vi "UI Limit Sensor.vi"(8 "error in":errorcluster) -> (0 "error out":errorcluster)   [LabVIEW 2019, in "Test.lvlib"]
uses:
  Test.lvlib
  Queues/Message Cluster.ctl
  Fluidic Process/SubVI/Fluidic Para.ctl
  <vilib>/Utility/file.llb/Write Delimited Spreadsheet (string).vi
  <vilib>/Utility/file.llb/Read Delimited Spreadsheet (string).vi
  Controller/Controller.lvlib
  Queues/Queues.lvlib
  Fluidic Process/Fluidic Process.lvlib
  Syringe Pump/NE-500/NE-500.lvlib
  Initialize/Initialize.lvlib
panel:
  out "Limit Sensor":bool
  in  "Stop Process":bool
  out "Remaining Time(s)":dbl
  out "Total Process":string
  out "Current Process":string
  out "Gauge":dbl(knob)=1.2869315802184793e-48 scale=0.0..100.0
  in  "Limit Sensor":bool
  in  "Back":bool
  # "/"
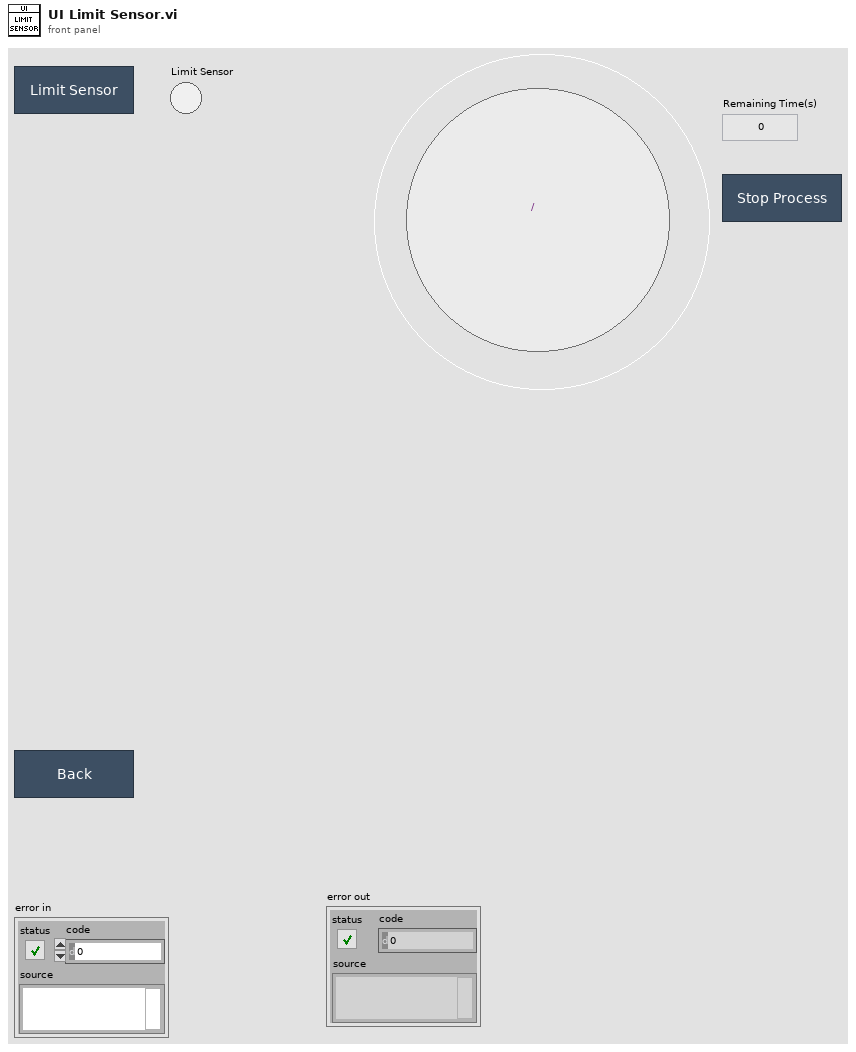
[diagram p1: front panel]
types:
  T1 = cluster{"Limit Sensor":refnum<queue>, "Limit Sensor Data":refnum<queue>}
  T2 = enum8{"Enabled", "Disabled", "Disabled and Grayed Out"}
  T3 = typedef "Fluidic Process.lvlib/Fluidic Para.ctl" = cluster{"Read Force Sensor":i32, "Read Regulator":i32, "Read Force Sensor?":bool, "Read Regulator?":bool, "Read Syringe Pump":i32, "Read Syringe Pump?":bool}
  T4 = typedef "Fluidic Process.lvlib/SEQ Data.ctl" = cluster{"Fluidic Process Done?":bool, "Current Process":i32, "Remaining Time":dbl, "Total Process":i32, "Air Sealing":bool, "Force Condition":bool}
  T5 = typedef "Initialize.lvlib/SEQ Data.ctl" = cluster{"Folder Path":path}
  T6 = typedef "NE-500.lvlib/SEQ Data.ctl" = cluster{"Status":string, "Initialize Done?":bool, "VI Refnum":refnum<vi>}
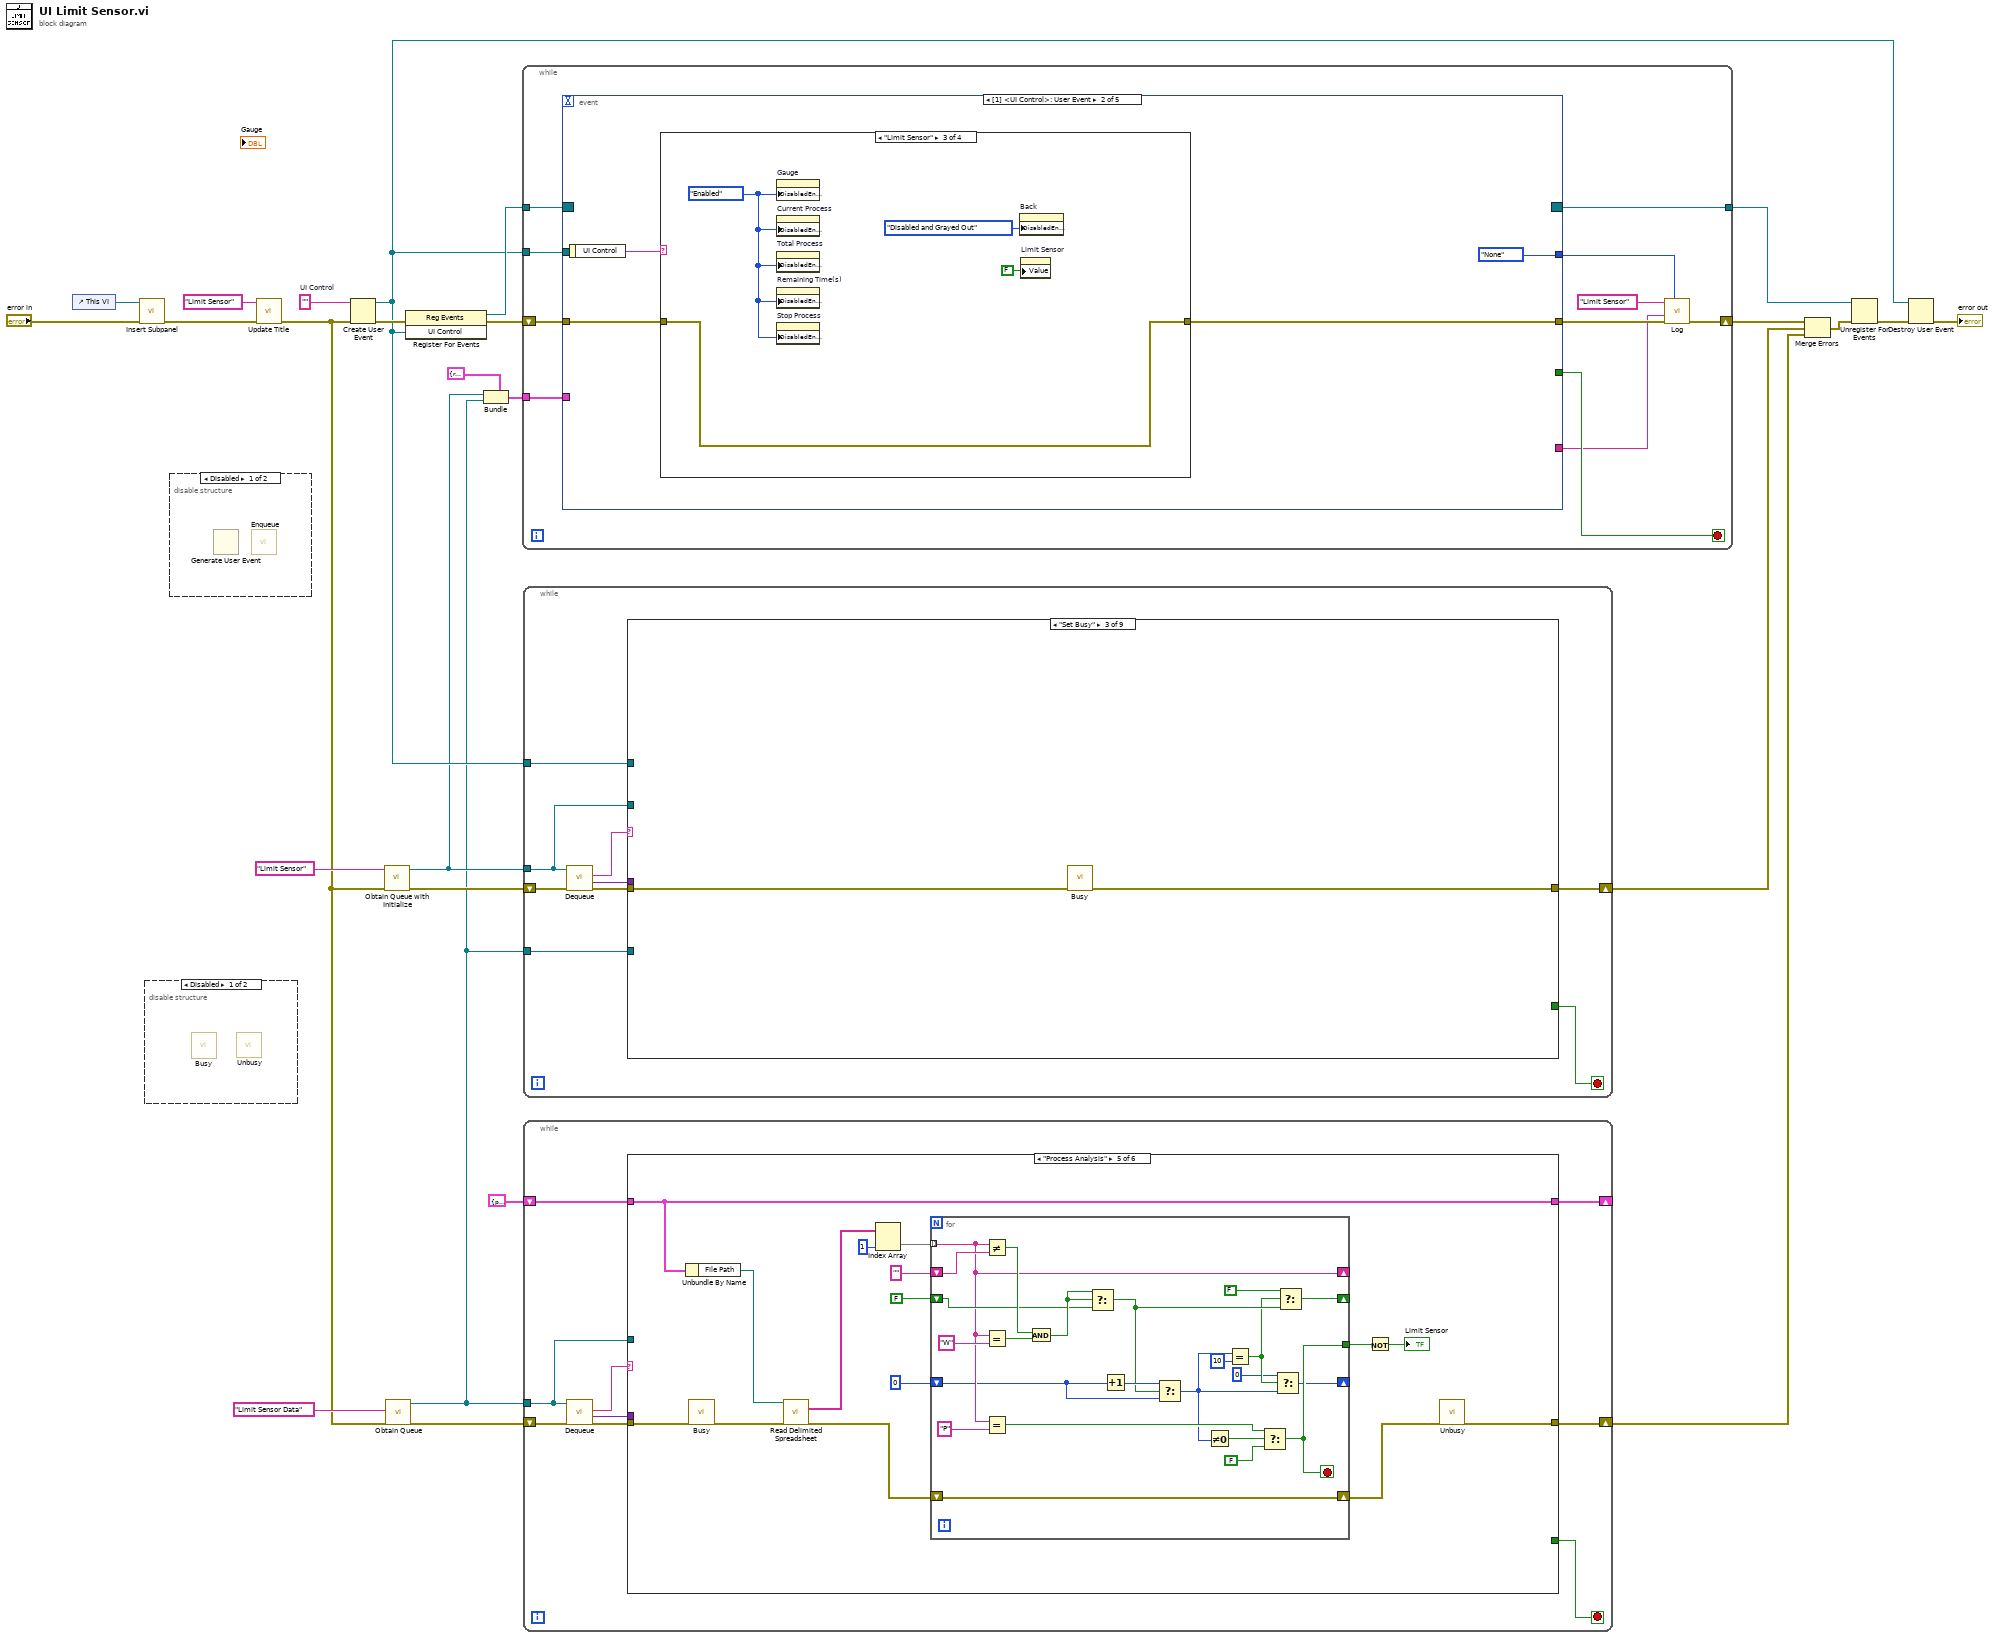
[diagram p0: block diagram]
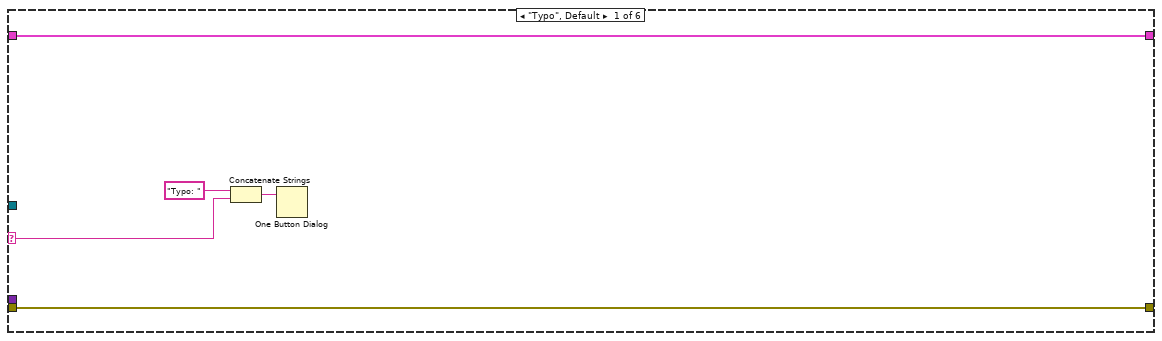
[diagram p3: hidden frame]
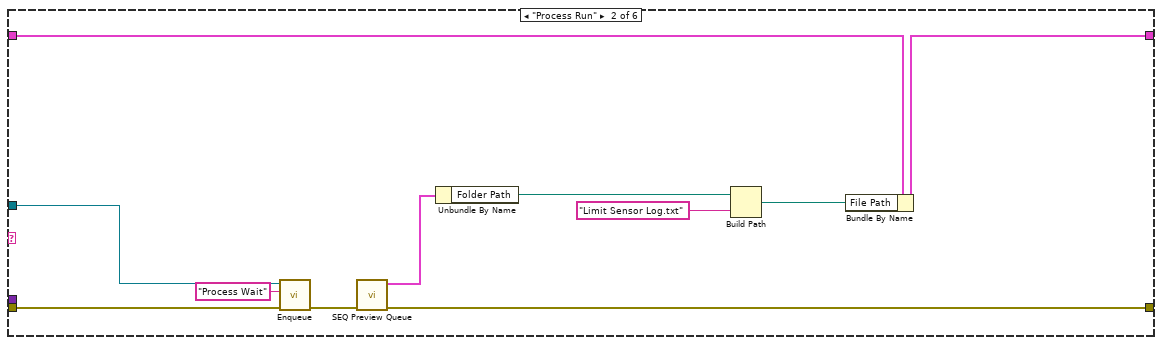
[diagram p4: hidden frame]
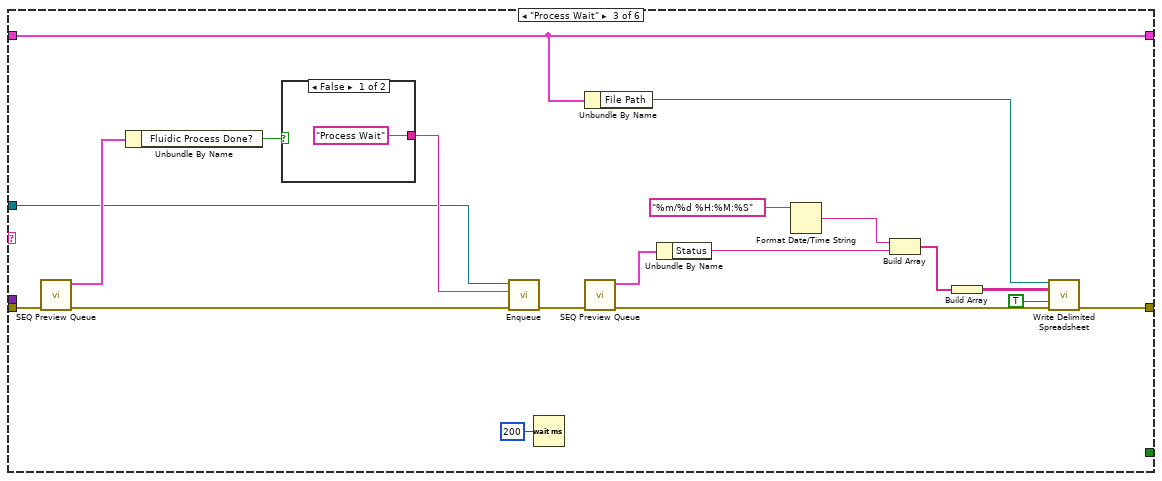
[diagram p5: hidden frame]
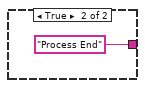
[diagram p6: hidden frame]
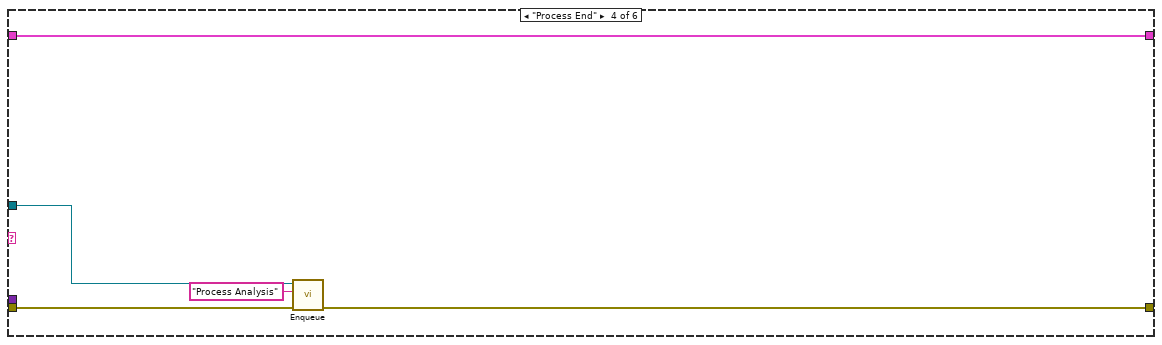
[diagram p7: hidden frame]
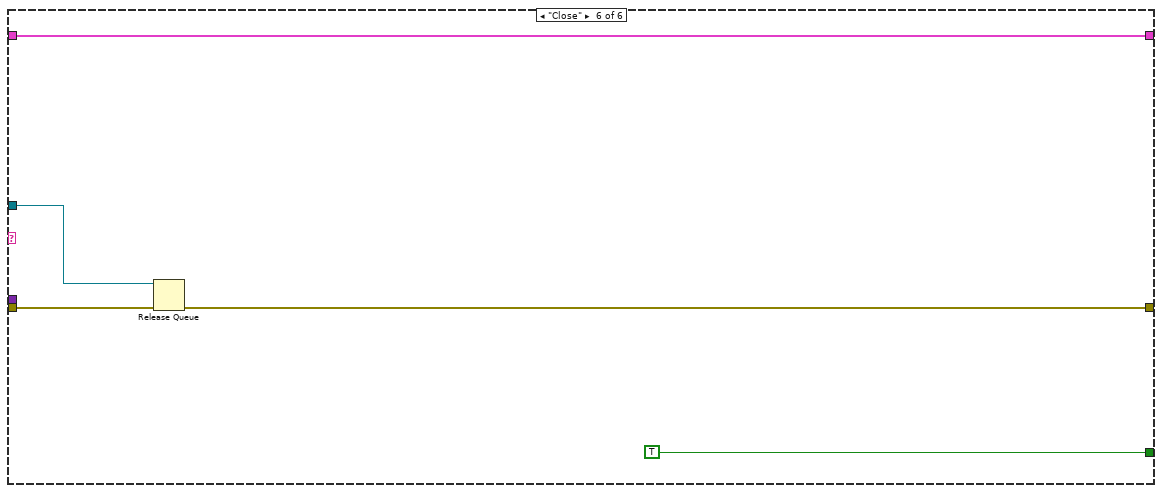
[diagram p8: hidden frame]
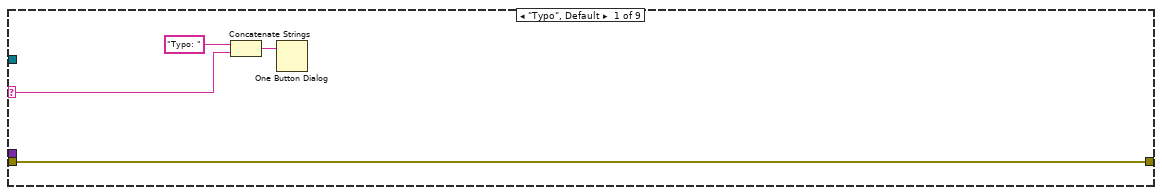
[diagram p10: hidden frame]
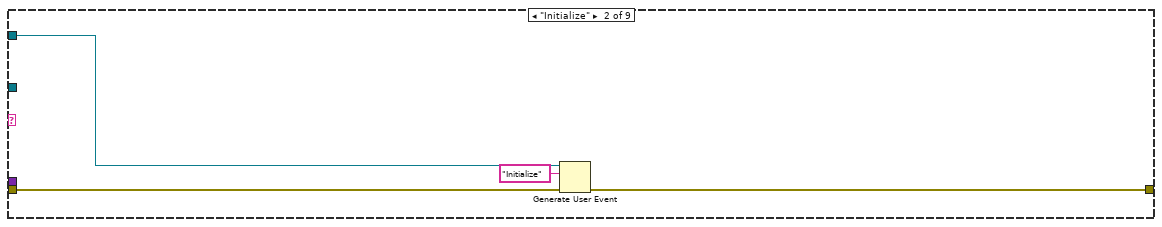
[diagram p11: hidden frame]
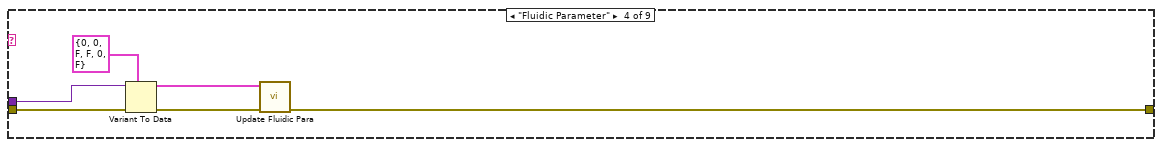
[diagram p12: hidden frame]
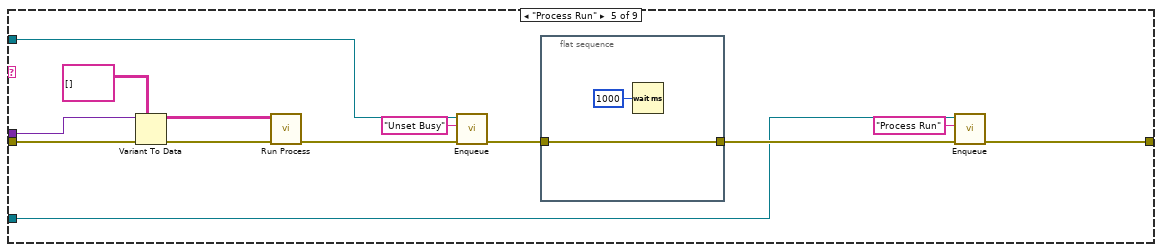
[diagram p13: hidden frame]
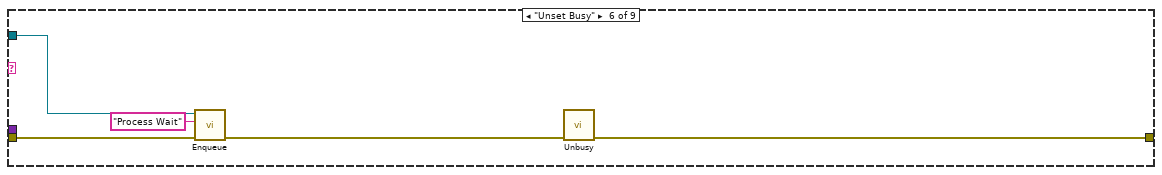
[diagram p14: hidden frame]
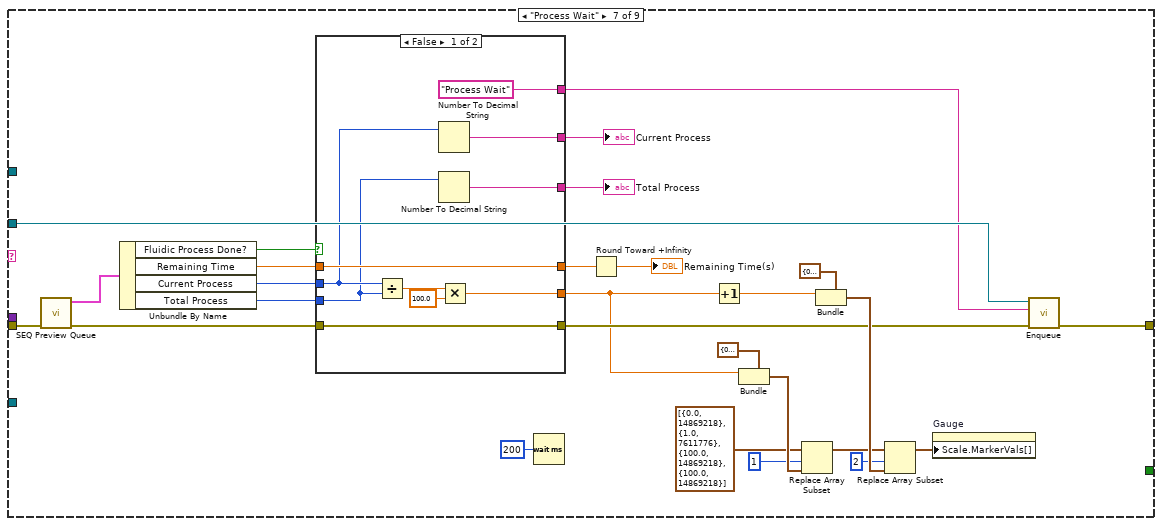
[diagram p15: hidden frame]
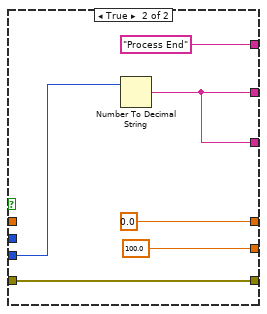
[diagram p16: hidden frame]
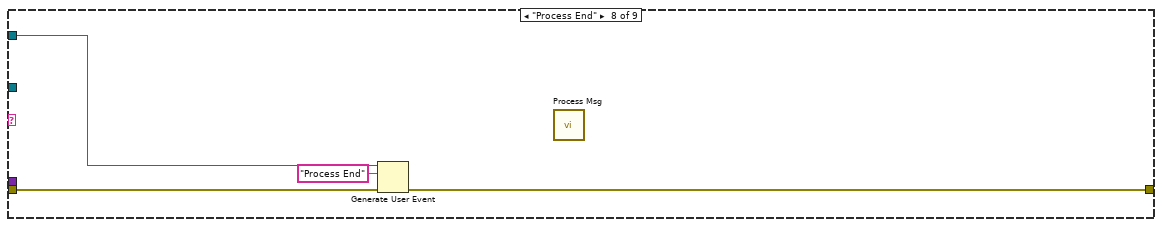
[diagram p17: hidden frame]
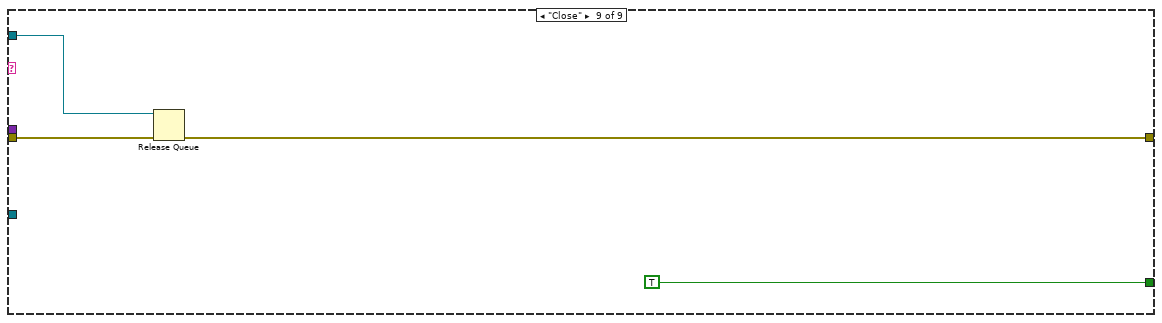
[diagram p18: hidden frame]
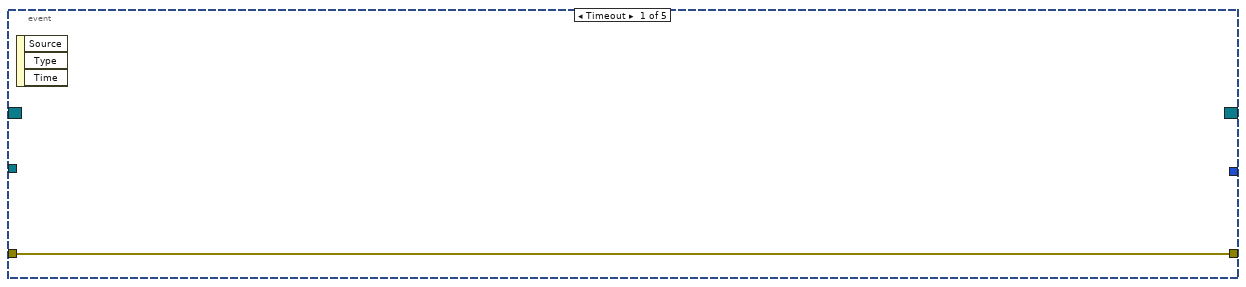
[diagram p19: hidden frame]
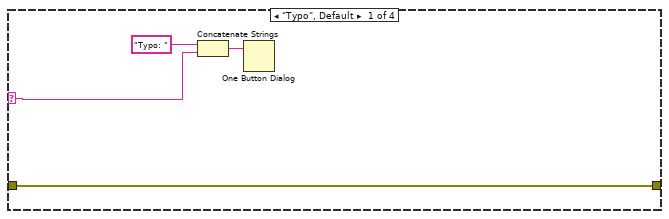
[diagram p20: hidden frame]
diagram:
  w16 = ""  # UI Control
  n1 = control-ref of="This VI"() -> (w15:refnum<vi>)
  n2 = call "Insert Subpanel.vi"("Error In"="error in", "VI Refnum"=w15) -> ("Error Out"=w4:errorcluster)  [unwired: 9 in]
  n3 = disable-structure shown="Disabled" {
    frame Disabled {
      n4 = call "Busy.vi"() -> ()  [unwired: 11 in, 1 out]
      n5 = call "Unbusy.vi"() -> ()  [unwired: 11 in, 1 out]
    }
    frame Enabled {
    }
  }
  n6 = disable-structure shown="Disabled" {
    frame Disabled {
      n7 = Generate User Event() -> ()  [unwired: 4 in, 2 out]
      n8 = call "Enqueue.vi"() -> ()  [unwired: 10 in, 2 out]
    }
    frame Enabled {
    }
  }
  n9 = call "Update Title.vi"("Error In"=w4, "Title"="Limit Sensor") -> ("Error Out"=w3:errorcluster)  [unwired: 9 in]
  n10 = Create User Event(user event datatype=w16, error in=w3) -> (user event=w14:refnum<user-event>, error out=w25:errorcluster)
  n11 = call "Obtain Queue with Initialize.vi"("Error In"=w3, "Queue Name"="Limit Sensor") -> ("Error Out"=w13:errorcluster, "Queue out"=w10:refnum<queue>)  [unwired: 8 in]
  n12 = call "Obtain Queue.vi"("Error In"=w3, "Queue Name"="Limit Sensor Data") -> ("Error Out"=w7:errorcluster, "queue out"=w1:refnum<queue>)  [unwired: 8 in]
  n13 = register-events(error in=w25, w14) -> (reference out=w23:refnum<event-registration>, error out=w24:errorcluster)  [unwired: 1 in]
  n14 = Bundle(cluster=T1 {"Limit Sensor"=refnum, "Limit Sensor Data"=refnum}, "Limit Sensor"=w10, "Limit Sensor Data"=w1) -> (w8:T1)
  n15 = while {
    tunnel: w23 -> [w35]
    shift-right: [w30] -> w21
    shift-left: w24 -> [w37]
    tunnel: [w34] -> w19
    tunnel: w14 -> [w33]
    tunnel: w8 -> [w32]
    stop <- w36 stop-if-true
    n16 = event shown="[1] <UI Control>: User Event" {
      selector: w35 -> [_ _ _ _ _]
      dyn-events: [_ _ _ _ _] -> w34
      timeout: _ -> [_ _ _ _ _]
      tunnel: w37 -> [w38 w42 w65 w90 w96]
      tunnel: [_ _ _ _ TRUE] -> w36
      tunnel: [w38 w40 w56 w89 w97] -> w31
      tunnel: w33 -> [_ _ w63 _ _]
      tunnel: w32 -> [_ _ w61 _ w95]
      tunnel: [_ enum16{"None", "Write"}."None" ("Action") enum16{"None", "Write"}."Write" ("Action") enum16{"None", "Write"}."Write" ("Action") enum16{"None", "Write"}."Write" ("Action")] -> w28
      tunnel: [_ _ w58 w86 w91] -> w27
      event Timeout {
        n17 = event-data() -> ()  [unwired: 1 in, 3 out]
      }
      event User Event {
        n18 = event-data() -> ("UI Control"=w41:string)  [unwired: 1 in]
        n19 = case shown="\"Limit Sensor\"" w41 {
          selector: w41 -> [w44 _ _ _]
          tunnel: w42 -> [w43 w48 w52 w55]
          tunnel: [w43 w48 w52 w55] -> w40
          frame "Typo", Default {
            n20 = Concatenate Strings("Typo: " ("string"), w44) -> (w45:string)
            n21 = One Button Dialog(message=w45) -> ()  [unwired: 1 in, 1 out]
          }
          frame "Initialize" {
            w47 = T2."Disabled and Grayed Out" ("Disabled")
            n22 = property on="Gauge" class="Knob (strict)"("DisabledEnum"=w47) -> ()  [unwired: 2 in, 2 out]
            n23 = property on="Current Process" class="Str"("DisabledEnum"=w47) -> ()  [unwired: 2 in, 2 out]
            n24 = property on="Total Process" class="Str"("DisabledEnum"=w47) -> ()  [unwired: 2 in, 2 out]
            n25 = property on="Remaining Time(s)" class="DigNum (strict)"("DisabledEnum"=w47) -> ()  [unwired: 2 in, 2 out]
            n26 = property on="Stop Process" class="Bool"("DisabledEnum"=w47) -> ()  [unwired: 2 in, 2 out]
          }
          frame "Limit Sensor" {
            w51 = T2."Enabled" ("Disabled")
            n27 = property on="Gauge" class="Knob (strict)"("DisabledEnum"=w51) -> ()  [unwired: 2 in, 2 out]
            n28 = property on="Current Process" class="Str"("DisabledEnum"=w51) -> ()  [unwired: 2 in, 2 out]
            n29 = property on="Total Process" class="Str"("DisabledEnum"=w51) -> ()  [unwired: 2 in, 2 out]
            n30 = property on="Remaining Time(s)" class="DigNum (strict)"("DisabledEnum"=w51) -> ()  [unwired: 2 in, 2 out]
            n31 = property on="Stop Process" class="Bool"("DisabledEnum"=w51) -> ()  [unwired: 2 in, 2 out]
            n32 = property on="Back" class="Bool"("DisabledEnum"=T2."Disabled and Grayed Out" ("Disabled")) -> ()  [unwired: 2 in, 2 out]
            n33 = property on="Limit Sensor" class="Bool (strict)"("Value"=FALSE ("Limit Sensor")) -> ()  [unwired: 2 in, 2 out]
          }
          frame "Process End" {
            w54 = T2."Disabled and Grayed Out" ("Disabled")
            n34 = property on="Gauge" class="Knob (strict)"("DisabledEnum"=w54) -> ()  [unwired: 2 in, 2 out]
            n35 = property on="Current Process" class="Str"("DisabledEnum"=w54) -> ()  [unwired: 2 in, 2 out]
            n36 = property on="Total Process" class="Str"("DisabledEnum"=w54) -> ()  [unwired: 2 in, 2 out]
            n37 = property on="Remaining Time(s)" class="DigNum (strict)"("DisabledEnum"=w54) -> ()  [unwired: 2 in, 2 out]
            n38 = property on="Stop Process" class="Bool"("DisabledEnum"=w54) -> ()  [unwired: 2 in, 2 out]
            n39 = property on="Back" class="Bool"("DisabledEnum"=T2."Enabled" ("Disabled")) -> ()  [unwired: 2 in, 2 out]
          }
        }
      }
      event "Limit Sensor": Value Change {
        n40 = event-data() -> ("CtlRef"=w59:refnum<vi>)  [unwired: 1 in]
        n41 = Unbundle By Name(w61) -> ("Limit Sensor"=w60:refnum<queue>)
        n42 = property class="Bool"(reference=w59) -> ("Label.Text"=w58:string)  [unwired: 1 in, 2 out]
        n43 = Generate User Event(user event=w63, event data cluster="Limit Sensor" ("event data"), error in=w65) -> (error out=w64:errorcluster)  [unwired: 1 in, 1 out]
        n44 = disable-structure shown="RUN_TIME_ENGINE==True" {
          disable-tunnel: [w75 w78] -> w73
          frame condition #0 (active) {
            n45 = call <vilib>:"Application Directory.vi"() -> ("Application Directory"=w77:path)
            n46 = Build Path(base path=w77, name or relative path="Fluidic Process\\File\\Limit Sensor.txt") -> (appended path=w75:path)
          }
          frame condition #1 {
            n47 = call <vilib>:"Application Directory.vi"() -> ("Application Directory"=w80:path)
            n48 = Build Path(base path=w80, name or relative path="data\\File\\Limit Sensor.txt") -> (appended path=w78:path)
          }
        }
        n49 = call-poly <vilib>:"Read Delimited Spreadsheet.vi"("file path (dialog if empty)"=w73, "error in (no error)"=w64) -> ("all rows"=w72:string[][], "error out"=w74:errorcluster)  [unwired: 8 in, 4 out]
        n50 = To Variant(anything=T3 {"Read Force Sensor"=0, "Read Regulator"=0, "Read Force Sensor?"=FALSE, "Read Regulator?"=FALSE, "Read Syringe Pump"=0, "Read Syringe Pump?"=FALSE} ("Cluster")) -> (Variant=w68:variant)
        n51 = To Variant(anything=w72) -> (Variant=w70:variant)
        n52 = Build Array(variant, w68, w70) -> (w67:variant[])
        n53 = for {
          shift-right: [w84] -> w56
          shift-left: w74 -> [w85]
          tunnel: string[] ["Set Busy", "Fluidic Parameter", "Process Run"] -> [w83] mode=indexing
          tunnel: w67 -> [w82] mode=indexing
          tunnel: w60 -> [w81]
          n54 = call "Enqueue.vi"("Error In"=w85, "Data"=w82, "State"=w83, "Queue in"=w81) -> ("Error Out"=w84:errorcluster)  [unwired: 6 in, 1 out]
        }
      }
      event "Stop Process": Value Change {
        n55 = event-data() -> ("CtlRef"=w87:refnum<vi>)  [unwired: 1 in]
        n56 = property class="Bool"(reference=w87) -> ("Label.Text"=w86:string)  [unwired: 1 in, 2 out]
        n57 = call "Stop Process.vi"("Error In"=w90) -> ("Error Out"=w89:errorcluster)  [unwired: 10 in]
      }
      event "Back": Value Change {
        n58 = event-data() -> ("CtlRef"=w92:refnum<vi>)  [unwired: 1 in]
        n59 = Cluster To Array(cluster=w95) -> (array=w94:refnum<queue>[])
        n60 = property class="Bool"(reference=w92) -> ("Label.Text"=w91:string)  [unwired: 1 in, 2 out]
        n61 = for {
          shift-right: [w102] -> w97
          shift-left: w96 -> [w100]
          tunnel: w94 -> [w99] mode=indexing
          n62 = call "Enqueue.vi"("Error In"=w100, "State"="Close", "Queue in"=w99) -> ("Error Out"=w102:errorcluster)  [unwired: 7 in, 1 out]
        }
      }
    }
    n63 = call "Log.vi"("Action"=w28, "error in"=w31, "Description"=w27, "Page Name"="Limit Sensor") -> ("error out"=w30:errorcluster)  [unwired: 7 in]
  }
  n64 = while {
    tunnel: w10 -> [w108]
    shift-right: [w106] -> w20
    shift-left: w13 -> [w111]
    tunnel: w14 -> [w105]
    tunnel: w1 -> [w103]
    stop <- w104 stop-if-true
    n65 = call "Dequeue.vi"("Error In"=w111, "Queue in"=w108) -> ("Error Out"=w107:errorcluster, "Data"=w109:variant, "State"=w110:string)  [unwired: 6 in, 1 out]
    n66 = case shown="\"Set Busy\"" w110 {
      selector: w110 -> [w113 _ _ _ _ _ _ _ _]
      tunnel: w109 -> [_ _ _ w126 w139 _ _ _ _]
      tunnel: w108 -> [_ _ _ _ w134 w146 w152 _ w196]
      tunnel: w107 -> [w112 w119 w121 w127 w140 w147 w174 w194 w198]
      tunnel: [_ _ _ _ _ _ _ _ TRUE] -> w104
      tunnel: [w112 w118 w120 w122 w130 w143 w158 w193 w197] -> w106
      tunnel: w105 -> [_ w117 _ _ _ _ _ w192 _]
      tunnel: w103 -> [_ _ _ _ w129 _ _ _ _]
      frame "Typo", Default {
        n67 = Concatenate Strings("Typo: " ("string"), w113) -> (w115:string)
        n68 = One Button Dialog(message=w115) -> ()  [unwired: 1 in, 1 out]
      }
      frame "Initialize" {
        n69 = Generate User Event(user event=w117, event data cluster="Initialize" ("event data"), error in=w119) -> (error out=w118:errorcluster)  [unwired: 1 in, 1 out]
      }
      frame "Set Busy" {
        n70 = call "Busy.vi"("Error In"=w121) -> ("Error Out"=w120:errorcluster)  [unwired: 10 in]
      }
      frame "Fluidic Parameter" {
        n71 = Variant To Data(error in=w127, type=T3 {"Read Force Sensor"=0, "Read Regulator"=0, "Read Force Sensor?"=FALSE, "Read Regulator?"=FALSE, "Read Syringe Pump"=0, "Read Syringe Pump?"=FALSE} ("Cluster"), Variant=w126) -> (data=w123:T3, error out=w124:errorcluster)
        n72 = call "Update Fluidic Para.vi"("Error In"=w124, "Fluidic Para"=w123) -> ("Error Out"=w122:errorcluster)  [unwired: 9 in]
      }
      frame "Process Run" {
        n73 = Variant To Data(error in=w140, type=string[][] [] ("all rows"), Variant=w139) -> (data=w136:string[][], error out=w137:errorcluster)
        n74 = call "Run Process.vi"("Error In"=w137, "Fluidic Process in"=w136) -> ("Error Out"=w135:errorcluster)  [unwired: 9 in]
        n75 = call "Enqueue.vi"("Error In"=w135, "State"="Unset Busy", "Queue in"=w134) -> ("Error Out"=w132:errorcluster)  [unwired: 7 in, 1 out]
        n76 = flat-sequence {
          tunnel: w132 -> [w142]
          tunnel: [w142] -> w131
          frame #0 {
            n77 = Wait (ms)(milliseconds to wait=u32 1000) -> ()  [unwired: 1 out]
          }
        }
        n78 = call "Enqueue.vi"("Error In"=w131, "State"="Process Run", "Queue in"=w129) -> ("Error Out"=w130:errorcluster)  [unwired: 7 in, 1 out]
      }
      frame "Unset Busy" {
        n79 = call "Enqueue.vi"("Error In"=w147, "State"="Process Wait", "Queue in"=w146) -> ("Error Out"=w144:errorcluster)  [unwired: 7 in, 1 out]
        n80 = call "Unbusy.vi"("Error In"=w144) -> ("Error Out"=w143:errorcluster)  [unwired: 10 in]
      }
      frame "Process Wait" {
        n81 = call "SEQ Preview Queue.vi"("error in"=w174) -> ("error out"=w171:errorcluster, "SEQ Data"=w173:T4)  [unwired: 9 in]
        n82 = Unbundle By Name(w173) -> ("Fluidic Process Done?"=w172:bool, "Remaining Time"=w157:dbl, "Current Process"=w156:i32, "Total Process"=w155:i32)
        n83 = case shown="False" w172 {
          tunnel: w171 -> [w182 w190]
          tunnel: [w182 w190] -> w159
          tunnel: w157 -> [w181 _]
          tunnel: w156 -> [w179 _]
          tunnel: w155 -> [w178 w189]
          tunnel: [w181 0.0 ("Remaining Time")] -> w153
          tunnel: [w180 100.0] -> w154
          tunnel: [w177 w188] -> w151
          tunnel: [w176 w188] -> w150
          tunnel: ["Process Wait" "Process End"] -> w149
          frame False {
            n84 = Divide(x=w179, y=w178) -> (x/y=w184:dbl)
            n85 = Number To Decimal String(number=w179) -> (decimal integer string=w177:string)  [unwired: 1 in]
            n86 = Number To Decimal String(number=w178) -> (decimal integer string=w176:string)  [unwired: 1 in]
            n87 = Multiply(x=w184, y=100.0) -> (x*y=w180:dbl)
          }
          frame True {
            n88 = Number To Decimal String(number=w189) -> (decimal integer string=w188:string)  [unwired: 1 in]
          }
        }
        "Total Process" <- w150
        "Current Process" <- w151
        n89 = Wait (ms)(milliseconds to wait=u32 200) -> ()  [unwired: 1 out]
        n90 = Round Toward +Infinity(x=w153) -> (ceil(x): smallest int >= x=→"Remaining Time(s)":dbl)
        n91 = Increment(x=w154) -> (x+1=w167:dbl)
        n92 = Bundle(cluster=cluster{dbl, i32} {0.0, 7611776}, w154) -> (w166:cluster{dbl, i32})  [unwired: 1 in]
        n93 = Replace Array Subset(array=cluster{dbl, u32}[] [{0.0, 14869218}, {1.0, 7611776}, {100.0, 14869218}, {100.0, 14869218}] ("Scale.Marker Values[]"), new element=w166, index=1) -> (w168:cluster{dbl, u32}[])
        n94 = Bundle(cluster=cluster{dbl, i32} {0.0, 14869218}, w167) -> (w169:cluster{dbl, i32})  [unwired: 1 in]
        n95 = Replace Array Subset(array=w168, new element=w169, index=2) -> (w170:cluster{dbl, u32}[])
        n96 = property on="Gauge" class="Knob (strict)"("Scale.MarkerVals[]"=w170) -> ()  [unwired: 2 in, 2 out]
        n97 = call "Enqueue.vi"("Error In"=w159, "State"=w149, "Queue in"=w152) -> ("Error Out"=w158:errorcluster)  [unwired: 7 in, 1 out]
      }
      frame "Process End" {
        n98 = Generate User Event(user event=w192, event data cluster="Process End" ("event data"), error in=w194) -> (error out=w193:errorcluster)  [unwired: 1 in, 1 out]
        n99 = call "Process Msg"() -> ()  [unwired: 10 in, 2 out]
      }
      frame "Close" {
        n100 = Release Queue(queue=w196, error in (no error)=w198) -> (error out=w197:errorcluster)  [unwired: 1 in, 2 out]
      }
    }
  }
  n101 = while {
    tunnel: w1 -> [w204]
    shift-right: [w202] -> w11
    shift-left: w7 -> [w207]
    shift-right: [w199] -> _
    shift-left: cluster{"File Path":path} {"File Path"=path ""} -> [w200]
    stop <- w201 stop-if-true
    n102 = call "Dequeue.vi"("Error In"=w207, "Queue in"=w204) -> ("Error Out"=w203:errorcluster, "Data"=w205:variant, "State"=w206:string)  [unwired: 6 in, 1 out]
    n103 = case shown="\"Process Analysis\"" w206 {
      selector: w206 -> [w210 _ _ _ _ _]
      tunnel: w205 -> [_ _ _ _ _ _]
      tunnel: w204 -> [_ w223 w237 w247 _ w290]
      tunnel: w203 -> [w209 w214 w242 w248 w251 w292]
      tunnel: [_ _ _ _ _ TRUE] -> w201
      tunnel: [w209 w213 w224 w245 w252 w291] -> w202
      tunnel: w200 -> [w208 w221 w234 w249 w264 w288]
      tunnel: [w208 w219 w234 w249 w264 w288] -> w199
      frame "Typo", Default {
        n104 = Concatenate Strings("Typo: " ("string"), w210) -> (w212:string)
        n105 = One Button Dialog(message=w212) -> ()  [unwired: 1 in, 1 out]
      }
      frame "Process Run" {
        n106 = call "Enqueue.vi"("Error In"=w214, "State"="Process Wait", "Queue in"=w223) -> ("Error Out"=w217:errorcluster)  [unwired: 7 in, 1 out]
        n107 = call "SEQ Preview Queue.vi"("error in"=w217) -> ("error out"=w213:errorcluster, "SEQ Data"=w216:T5)  [unwired: 9 in]
        n108 = Unbundle By Name(w216) -> ("Folder Path"=w215:path)
        n109 = Build Path(base path=w215, name or relative path="Limit Sensor Log.txt") -> (appended path=w218:path)
        n110 = Bundle By Name(cluster=w221, "File Path"=w218) -> (w219:cluster{"File Path":path})
      }
      frame "Process Wait" {
        n111 = call "SEQ Preview Queue.vi"("error in"=w242) -> ("error out"=w236:errorcluster, "SEQ Data"=w241:T4)  [unwired: 9 in]
        n112 = Unbundle By Name(w241) -> ("Fluidic Process Done?"=w240:bool)
        n113 = case shown="False" w240 {
          tunnel: ["Process Wait" "Process End"] -> w238
          frame False {
          }
          frame True {
          }
        }
        n114 = call "Enqueue.vi"("Error In"=w236, "State"=w238, "Queue in"=w237) -> ("Error Out"=w235:errorcluster)  [unwired: 7 in, 1 out]
        n115 = Wait (ms)(milliseconds to wait=u32 200) -> ()  [unwired: 1 out]
        n116 = Unbundle By Name(w234) -> ("File Path"=w226:path)
        n117 = call "SEQ Preview Queue.vi"("error in"=w235) -> ("error out"=w225:errorcluster, "SEQ Data"=w233:T6)  [unwired: 9 in]
        n118 = Unbundle By Name(w233) -> ("Status"=w227:string)
        n119 = Format Date/Time String(time format string (%c)="%m/%d %H:%M:%S") -> (date/time string=w231:string)  [unwired: 2 in]
        n120 = Build Array(w231, w227) -> (w230:string[])
        n121 = Build Array(w230) -> (w232:string[][])
        n122 = call-poly <vilib>:"Write Delimited Spreadsheet.vi"("file path (dialog if empty)"=w226, "2D data"=w232, "append to file? (new file:F)"=TRUE, "error in (no error)"=w225) -> ("error out"=w224:errorcluster)  [unwired: 10 in, 1 out]
      }
      frame "Process End" {
        n123 = call "Enqueue.vi"("Error In"=w248, "State"="Process Analysis", "Queue in"=w247) -> ("Error Out"=w245:errorcluster)  [unwired: 7 in, 1 out]
      }
      frame "Process Analysis" {
        n124 = Unbundle By Name(w264) -> ("File Path"=w263:path)
        n125 = call "Busy.vi"("Error In"=w251) -> ("Error Out"=w250:errorcluster)  [unwired: 10 in]
        n126 = call-poly <vilib>:"Read Delimited Spreadsheet.vi"("file path (dialog if empty)"=w263, "error in (no error)"=w250) -> ("all rows"=w262:string[][], "error out"=w256:errorcluster)  [unwired: 8 in, 4 out]
        n127 = Index Array(array=w262, index (col)=1 ("disabled index (col)")) -> (element=w260:string[])  [unwired: 1 in]
        n128 = for {
          tunnel: w260 -> [w274] mode=indexing
          shift-right: [w274] -> _
          shift-left: "" -> [w284]
          shift-right: [w279] -> _
          shift-left: FALSE -> [w282]
          shift-right: [w267] -> _
          shift-left: 0 -> [w271]
          tunnel: [w275] -> w254
          shift-right: [w265] -> w253
          shift-left: w256 -> [w265]
          stop <- w275 stop-if-true
          n129 = Not Equal?(x=w274, y=w284) -> (x != y?=w286:bool)
          n130 = Equal?(x=w274, y="W") -> (x = y?=w285:bool)
          n131 = Equal?(x=w274, y="P") -> (x = y?=w272:bool)
          n132 = And(x=w286, y=w285) -> (x .and. y?=w283:bool)
          n133 = Select(t=w283, s=w283, f=w282) -> (s? t:f=w277:bool)
          n134 = Increment(x=w271) -> (x+1=w281:i32)
          n135 = Select(t=w281, s=w277, f=w271) -> (s? t:f=w268:i32)
          n136 = Not Equal To 0?(x=w268) -> (x != 0?=w270:bool)
          n137 = Equal?(x=w268, y=10) -> (x = y?=w269:bool)
          n138 = Select(t=w272, s=w270, f=FALSE) -> (s? t:f=w275:bool)
          n139 = Select(t=0, s=w269, f=w268) -> (s? t:f=w267:i32)
          n140 = Select(t=FALSE, s=w269, f=w277) -> (s? t:f=w279:bool)
        }
        n141 = Not(x=w254) -> (.not. x?=→"Limit Sensor":bool)
        n142 = call "Unbusy.vi"("Error In"=w253) -> ("Error Out"=w252:errorcluster)  [unwired: 10 in]
      }
      frame "Close" {
        n143 = Release Queue(queue=w290, error in (no error)=w292) -> (error out=w291:errorcluster)  [unwired: 1 in, 2 out]
      }
    }
  }
  n144 = Merge Errors(w21, w20, w11) -> (w18:errorcluster)
  n145 = Unregister For Events(event registration refnum=w19, error in=w18) -> (error out=w17:errorcluster)
  n146 = Destroy User Event(user event=w14, error in=w17) -> (error out=→"error out":errorcluster)
